vi "Open.vi"(7 "SPI Channel (0)":u8, 8 "Error In":errorcluster, 11 "LINX Ref":T1) -> (0 "Error Out":errorcluster, 2 "Actual Clock Frequency":u32, 3 "LINX Resource":T1)   [LabVIEW 2014, in "LMH-LINX.lvlib" / "PmodMIC3.lvlib"]
doc: "Open the SPI channel and initialize the PmodMIC3."
uses:
  PmodMIC3.lvlib
  Private/Type Defs/LINX Ref.ctl
  Private/Type Defs/Platform.ctl
  Private/Type Defs/Interface.ctl
  Private/Device/Type Defs/LINX Device Config.ctl
  Private/Device/Type Defs/TCP Config.ctl
  Private/Device/Type Defs/Channels.ctl
  Private/Type Defs/Peripherals/SPI/SPI Configuration.ctl
  Private/Type Defs/Peripherals/SPI/SPI Bit Order.ctl
  Private/Type Defs/Peripherals/SPI/SPI Mode.ctl
  LMH-LINX.lvlib
  Private/Device/Device.lvlib
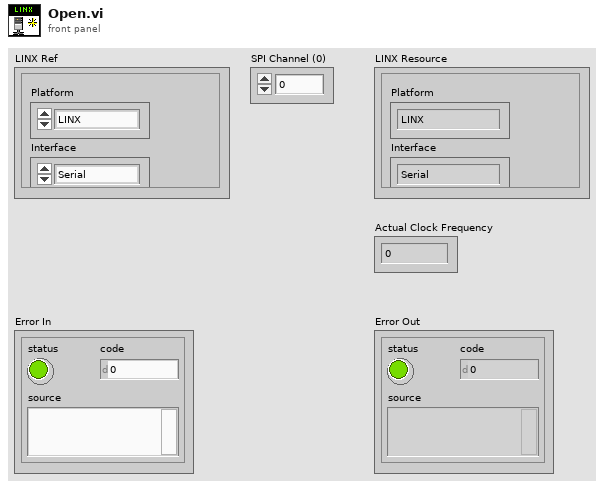
[diagram p1: front panel]
types:
  T1 = typedef "LMH-LINX.lvlib/LINX Ref.ctl" = cluster{"Platform":T2, "Interface":T3, "LINX Device Config":T4}
  T2 = typedef "LMH-LINX.lvlib/Platform.ctl" = enum16{"LINX", "myRIO"}
  T3 = typedef "LMH-LINX.lvlib/Interface.ctl" = enum16{"Serial", "TCP"}
  T4 = typedef "LMH-LINX.lvlib/Device.lvlib/LINX Device Config.ctl" = cluster{"Interface":T3, "COM Port":refnum<visa-resource-name>, "TCP Configuration":T5, "Device Family":u8, "Device ID":u8, "Device Name":string, "TCP Ref":refnum<k5>, "Channels":T6}
  T5 = typedef "LMH-LINX.lvlib/Device.lvlib/TCP Config.ctl" = cluster{"IP Address":string, "Port":u16}
  T6 = typedef "LMH-LINX.lvlib/Channels.ctl" = cluster{"DI":u8[], "DO":u8[], "AI":u8[], "AO":u8[], "PWM":u8[], "QE":u8[], "UART":u8[], "I2C 2":u8[], "SPI":u8[], "CAN":u8[], "Servo":u8[], "AI Ref (V)":dbl, "AO Ref (V)":dbl, "AO Resolution (Bits)":u8}
  T7 = typedef "LMH-LINX.lvlib/SPI Configuration.ctl" = cluster{"Clock Frequency":u32, "Bit Order":T8, "SPI Mode":T9}
  T8 = typedef "LMH-LINX.lvlib/SPI Bit Order.ctl" = enum8{"LSb First", "MSb First"}
  T9 = typedef "LMH-LINX.lvlib/SPI Mode.ctl" = enum8{"Mode 0", "Mode 1", "Mode 2", "Mode 3"}
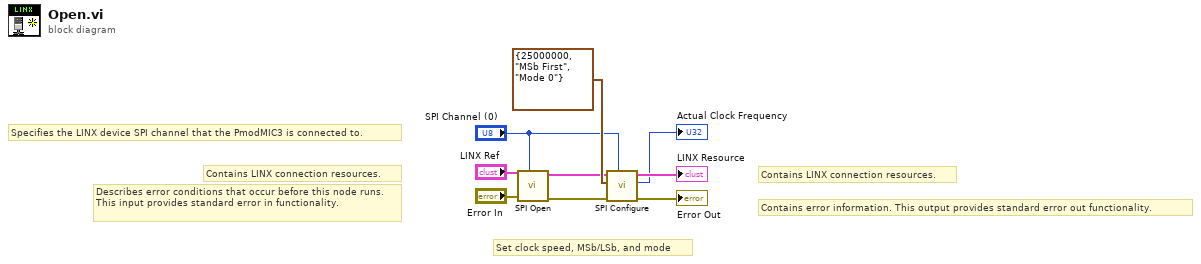
[diagram p0: block diagram]
diagram:
  # "Specifies the LINX device SPI channel that the PmodMIC3 is connected to."
  # "Contains LINX connection resources."
  # "Contains error information. This output provides standard error out functionality."
  # "Contains LINX connection resources."
  # "Describes error conditions that occur before this node runs. This input provides standard error in functionality."
  # "Set clock speed, MSb/LSb, and mode"
  n1 = call "SPI Open.vi"("SPI Channel (0)"="SPI Channel (0)", "Error In"="Error In", "LINX Resource"="LINX Ref") -> ("Error Out"=w4:errorcluster, "LINX Resource"=w3:T1)  [unwired: 7 in]
  n2 = call "SPI Configure.vi"("SPI Channel (0)"="SPI Channel (0)", "Error In"=w4, "SPI Configuration"=T7 {"Clock Frequency"=25000000, "Bit Order"=enum."MSb First", "SPI Mode"=enum."Mode 0"}, "LINX Resource"=w3) -> ("Error Out"=→"Error Out":errorcluster, "Actual Clock Frequency"=→"Actual Clock Frequency":u32, "LINX Resource"=→"LINX Resource":T1)  [unwired: 5 in]
